vi "Save Wordlist.vi"() -> ()   [LabVIEW 2024]
uses:
  2915c480-1779-4c6d-b6d9-cdf4db356fd9.vi
  Libraries/Wordle Engine/Wordle Engine.lvlib
panel:
  out "error out":errorcluster
  in  "# Words":i32=500
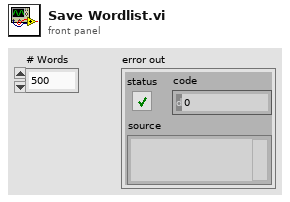
[diagram p1: front panel]
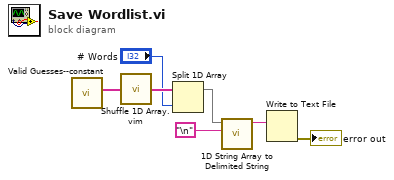
[diagram p0: block diagram]
diagram:
  n1 = call "Valid Guesses--constant.vi"() -> ("Valid Guesses (array)"=w7:string[])  [unwired: 10 in, 1 out]
  n2 = call "Shuffle 1D Array.vim"("array"=w7) -> ("shuffled array"=w6:string[])  [unwired: 4 in]
  n3 = Split 1D Array(array=w6, index="# Words") -> (first subarray=w4:string[])  [unwired: 1 out]
  n4 = call <vilib>:"1D String Array to Delimited String.vi"("delimiter"="\n", "string array"=w4) -> ("delimited string"=w2:string)  [unwired: 9 in]
  n5 = Write to Text File(text=w2) -> (error out=→"error out":errorcluster)  [unwired: 3 in, 2 out]
